vi "event_analyzer.vi"(6 "EventAction":T1, 8 "error in (no error)":errorcluster) -> (0 "error out":errorcluster, 3 "Event Registration Refnum":refnum<event-registration>)   [LabVIEW 2020]
uses:
  #typedefs/#typedef_enum_EventActions.ctl
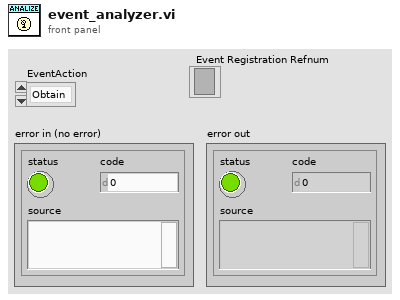
[diagram p1: front panel]
types:
  T1 = typedef "#typedef_enum_EventActions.ctl" = enum16{"Obtain", "GetRef", "Generate", "Destroy"}
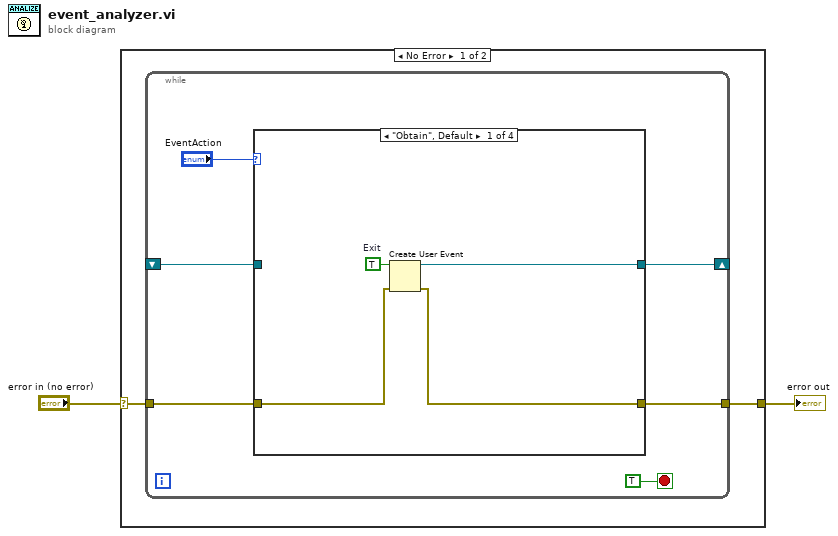
[diagram p0: block diagram]
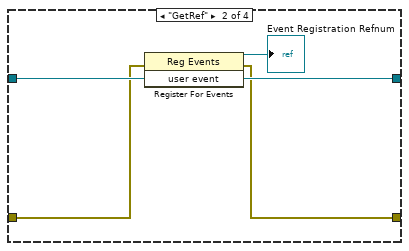
[diagram p2: hidden frame]
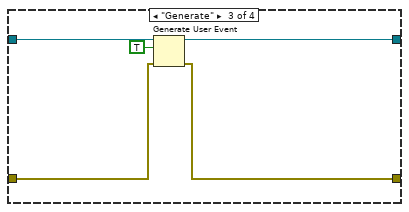
[diagram p3: hidden frame]
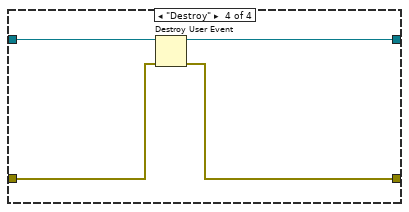
[diagram p4: hidden frame]
diagram:
  n1 = case shown="No Error" "error in (no error)" {
    selector: "error in (no error)" -> [w4 w27]
    tunnel: [w3 w27] -> w1
    frame No Error {
      n2 = while {
        shift-right: [w7] -> _
        shift-left: _ -> [w6]
        tunnel: w4 -> [w9]
        tunnel: [w8] -> w3
        stop <- TRUE stop-if-true
        n3 = case shown="\"Obtain\", Default" "EventAction" {
          tunnel: w9 -> [w13 w16 w20 w26]
          tunnel: [w12 w15 w19 w25] -> w8
          tunnel: [w11 w18 w22 w24] -> w7
          tunnel: w6 -> [_ w18 w23 w24]
          frame "Obtain", Default {
            w14 = TRUE  # Exit
            n4 = Create User Event(user event datatype=w14, error in=w13) -> (user event=w11:refnum<user-event>, error out=w12:errorcluster)
          }
          frame "GetRef" {
            n5 = register-events(error in=w16, w18) -> (reference out=→"Event Registration Refnum":refnum<event-registration>, error out=w15:errorcluster)  [unwired: 1 in]
          }
          frame "Generate" {
            n6 = Generate User Event(user event=w23, event data cluster=TRUE ("event data"), error in=w20) -> (user event out=w22:refnum<user-event>, error out=w19:errorcluster)  [unwired: 1 in]
          }
          frame "Destroy" {
            n7 = Destroy User Event(user event=w24, error in=w26) -> (error out=w25:errorcluster)
          }
        }
      }
    }
    frame Error {
    }
  }
  "error out" <- w1
